vi "Parse Notifier Name.vi"(7 "Notifier Name":string) -> (4 "Device Type":string, 8 "Function":string, 15 "Company":string)   [LabVIEW 2020]
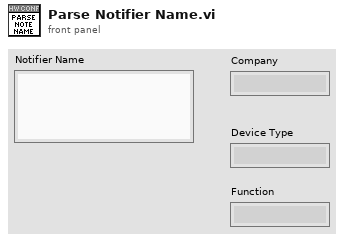
[diagram p1: front panel]
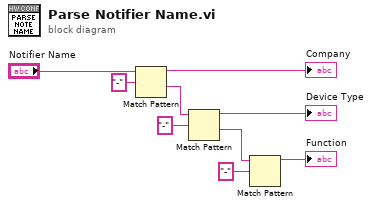
[diagram p0: block diagram]
diagram:
  n1 = Match Pattern(string="Notifier Name", regular expression="-") -> (before substring=→"Company":string, after substring=w5:string)  [unwired: 1 in, 2 out]
  n2 = Match Pattern(string=w5, regular expression="-") -> (before substring=→"Device Type":string, after substring=w2:string)  [unwired: 1 in, 2 out]
  n3 = Match Pattern(string=w2, regular expression="-") -> (before substring=→"Function":string)  [unwired: 1 in, 3 out]
